vi "SetNumThreads.vi"(8 "error in":errorcluster, 11 "nThreads":i32) -> (0 "error out":errorcluster)   [LabVIEW 2020, in "OpenLvVision_OpenCv.lvlib"]
doc: "OpenCV will try to set the number of threads for the next parallel region.\n\nIf threads == 0, OpenCV will disable threading optimizations and run all it's functions sequentially. Passing threads < 0 will reset threads number to system default."
uses:
  OpenLvVision_OpenCv.lvlib
  Dlls/OlvOpenCvWrapper.dll
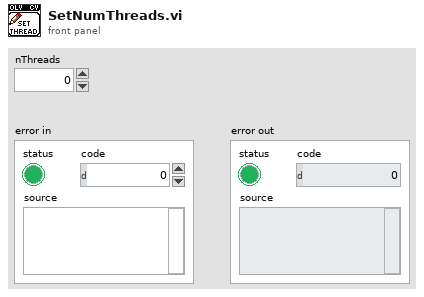
[diagram p1: front panel]
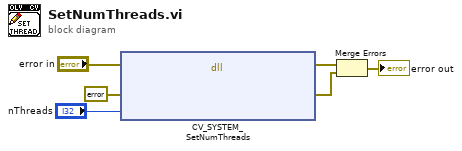
[diagram p0: block diagram]
diagram:
  n1 = dll-call lib="C:/Users/lukas/Downloads/OpenLvVision_OpenCv/SourceCode/LabView/OpenLvVision_OpenCv/Dlls/OlvOpenCvWrapper.dll" fn="CV_SYSTEM_SetNumThreads"(error in="error in", "Error"=errorcluster {"status"=FALSE, "code"=0, "source"=""} ("error in"), "nThreads"="nThreads") -> (error out=w4:errorcluster, "Error"=w2:errorcluster)  [unwired: 4 in, 1 out]
  n2 = Merge Errors(w4, w2) -> (→"error out":errorcluster)
